vi "PDC_OpenDevice.vi"(8 "error in (no error)":errorcluster, 9 "InterfaceCode":u32, 10 "TmpDeviceNo":u32 format="%.0x", 11 "DeviceCode":u32) -> (0 "error out":errorcluster, 1 "DeviceNo":u32, 2 "ErrorCode":u32, 3 "ReturnValue":u32)   [LabVIEW 2015]
doc: "This VI opens and initializes the specified device."
uses:
  PDCLIB.dll
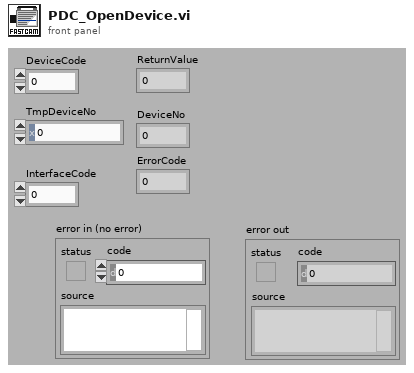
[diagram p1: front panel]
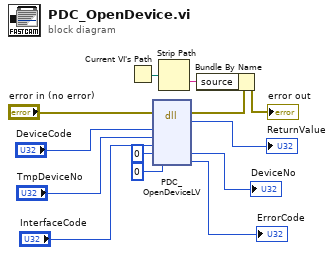
[diagram p0: block diagram]
diagram:
  n1 = Current VI's Path() -> (path=w3:path)
  n2 = dll-call lib="PDCLIB.dll" fn="PDC_OpenDeviceLV"(error in="error in (no error)", "nDeviceCode"="DeviceCode", "nTmpDeviceNo"="TmpDeviceNo", "nInterfaceCode"="InterfaceCode", "nDeviceNo"=u32 0, "pErrorCode"=u32 0) -> (error out=w2:errorcluster, "return type"=→"ReturnValue":u32, "nDeviceNo"=→"DeviceNo":u32, "pErrorCode"=→"ErrorCode":u32)  [unwired: 5 in, 1 out]
  n3 = Strip Path(path=w3) -> (name=w4:string)  [unwired: 1 out]
  n4 = Bundle By Name(cluster=w2, "source"=w4) -> (→"error out":errorcluster)
